vi "Create RPC Engine Loop Stop Notifier.vi"(8 "error in (no error)":errorcluster) -> (0 "error out":errorcluster)   [LabVIEW 2020, in "JSON-RPC Lib.lvlib" / "JSONRPC Server.lvclass"]
uses:
  JSONRPC Server.lvclass
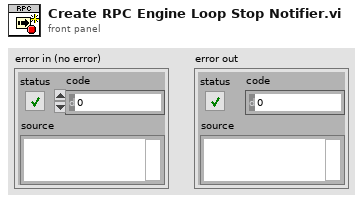
[diagram p1: front panel]
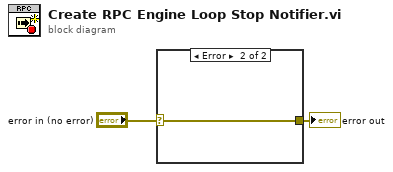
[diagram p0: block diagram]
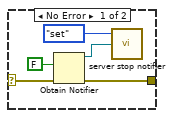
[diagram p2: hidden frame]
diagram:
  n1 = case shown="Error" "error in (no error)" {
    selector: "error in (no error)" -> [w4 w8]
    tunnel: [w5 w8] -> w2
    frame No Error {
      n2 = Obtain Notifier(notification data type=FALSE, error in (no error)=w4) -> (notifier out=w6:refnum<notifier>, error out=w5:errorcluster)  [unwired: 2 in, 1 out]
      n3 = call "server stop notifier.vi"("notifier in"=w6, "action"=enum16{"get", "set"}."set") -> ()  [unwired: 1 in, 1 out]
    }
    frame Error {
    }
  }
  "error out" <- w2
